vi "Ip-temp.vi"(2 "index":i32, 3 "row in":sgl[](array[numeric]), 4 "array in":sgl[][](array[numeric]), 5 "command":enum16{"get", "set", "clear", "add row"}(ring)) -> (0 "range":cluster{"min":sgl, "max":sgl}, 1 "array out":sgl[][](array[numeric]))   [LabVIEW 2013]
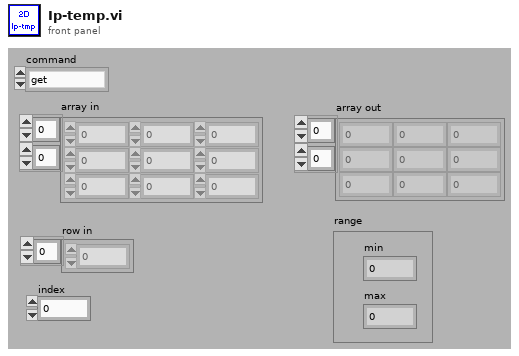
[diagram p1: front panel]
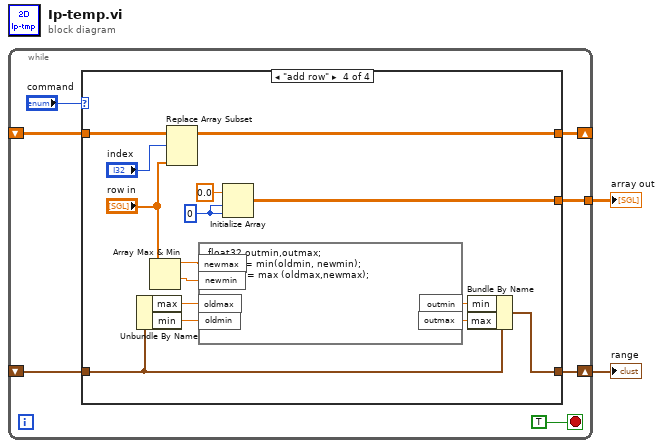
[diagram p0: block diagram]
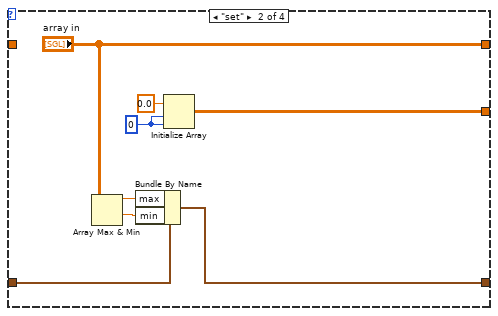
[diagram p3: hidden frame]
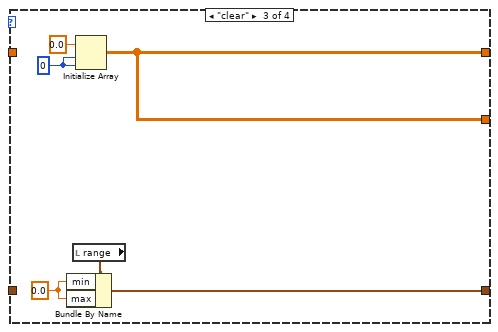
[diagram p4: hidden frame]
diagram:
  n1 = while {
    shift-right: [w7] -> _
    shift-left: _ -> [w8]
    tunnel: [w6] -> w2
    shift-right: [w5] -> w1
    shift-left: _ -> [w4]
    stop <- TRUE stop-if-true
    n2 = case shown="\"add row\"" "command" {
      tunnel: [w11 "array in" w23 w39] -> w7
      tunnel: w8 -> [w11 _ _ w40]
      tunnel: [w11 w17 w23 w35] -> w6
      tunnel: [w10 w12 w20 w26] -> w5
      tunnel: w4 -> [w10 w13 _ w27]
      frame "get", Default {
      }
      frame "set" {
        w18 = 0 ("dimension size")
        n3 = Array Max & Min(array="array in") -> (max value=w15:sgl, min value=w14:sgl)  [unwired: 2 out]
        n4 = Bundle By Name(cluster=w13, "max"=w15, "min"=w14) -> (w12:cluster{"min":sgl, "max":sgl})
        n5 = Initialize Array(sgl 0.0 ("element"), w18, w18) -> (w17:sgl[][])
      }
      frame "clear" {
        w21 = sgl 0.0 ("min")
        w24 = 0 ("dimension size")
        n6 = local read "range"() -> (w22:cluster{"min":sgl, "max":sgl})
        n7 = Bundle By Name(cluster=w22, "min"=w21, "max"=w21) -> (w20:cluster{"min":sgl, "max":sgl})
        n8 = Initialize Array(sgl 0.0 ("element"), w24, w24) -> (w23:sgl[][])
      }
      frame "add row" {
        w36 = 0 ("dimension size")
        n9 = Unbundle By Name(w27) -> ("max"=w31:sgl, "min"=w30:sgl)
        n10 = Array Max & Min(array="row in") -> (max value=w33:sgl, min value=w32:sgl)  [unwired: 2 out]
        n11 = Replace Array Subset(array=w40, new element="row in", index (row)="index") -> (w39:sgl[][])  [unwired: 1 in]
        n12 = formula code="float32 outmin,outmax;\noutmin = min(oldmin, newmin);\noutmax = max (oldmax,newmax);"("oldmin"=w30, "oldmax"=w31, "newmax"=w33, "newmin"=w32) -> ("outmin"=w29:sgl, "outmax"=w28:sgl)
        n13 = Initialize Array(sgl 0.0 ("element"), w36, w36) -> (w35:sgl[][])
        n14 = Bundle By Name(cluster=w27, "min"=w29, "max"=w28) -> (w26:cluster{"min":sgl, "max":sgl})
      }
    }
  }
  "array out" <- w2
  "range" <- w1
